vi "Persistent Read.vi"(4 "error in (no error)":errorcluster, 6 "Container State":T4, 7 "Display State In":T3) -> (0 "error out":errorcluster, 2 "Value":T1, 3 "Display State Out":T3)   [LabVIEW 2020, in "Waveform (G3).xctl"]
uses:
  Waveform (G3).xctl
  <vilib>/_xctls/Container State.ctl
  State.ctl
  Utility VIs/Controls/KRing/KRing.xctl
  Tone (G3)/Tone (G3).xctl
  Noise (G3)/Noise (G3).xctl
  Noise (G3)/Noise (G3) - Persistent.ctl
  Waveform (G3) - Persistent.ctl
  <vilib>/_xctls/XControlSupport.lvlib
panel:
  # "Replace the Value Indicator below with an Indicator of desired type.\nDo not remove this Indicator or the others from the connector pane. \nDo not change the connector pane pattern.\nThe Value Indicator should always be the second terminal from top on the output side in the connector pane."
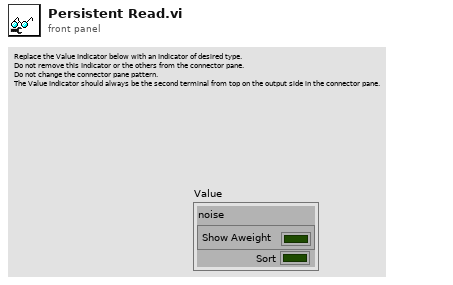
[diagram p1: front panel]
types:
  T1 = typedef "Waveform (G3).xctl/Waveform (G3) - Persistent.ctl" = cluster{"noise":T2, "Sort":bool}
  T2 = typedef "Noise (G3).xctl/Noise (G3) - Persistent.ctl" = cluster{"Show Aweight":bool}
  T3 = typedef "Waveform (G3).xctl/State.ctl" = cluster{"Waveform names":string[], "Valid":bool[], "enable menu":bool, "Controls":cluster{"Type ":refnum<vi>, "Tone ":refnum<vi>, "Noise":refnum<vi>}, "persistent":cluster{"noise":T2, "Sort":bool}, "multi":bool}
  T4 = typedef "XControlSupport.lvlib/Container State.ctl" = cluster{"Indicator?":bool, "Run Mode?":bool, " Refnum":refnum<vi>}
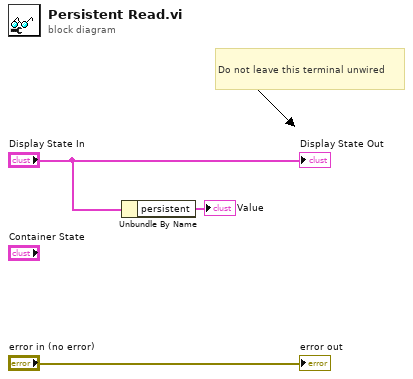
[diagram p0: block diagram]
diagram:
  # "Do not leave this terminal unwired"
  n1 = Unbundle By Name("Display State In") -> ("persistent"=→"Value":cluster{"noise":T2, "Sort":bool})
  "error out" <- "error in (no error)"
  "Display State Out" <- "Display State In"
